vi "insert_log_entry.vi"(8 "error in (no error)":errorcluster, 10 "message":string, 11 "GenericPlugin in":refnum<class "GenericComponent.lvclass">) -> (0 "error out":errorcluster, 3 "GenericPlugin out":refnum<class "GenericComponent.lvclass">)   [LabVIEW 2010, in "GenericComponent.lvclass"]
uses:
  GenericComponent.lvclass
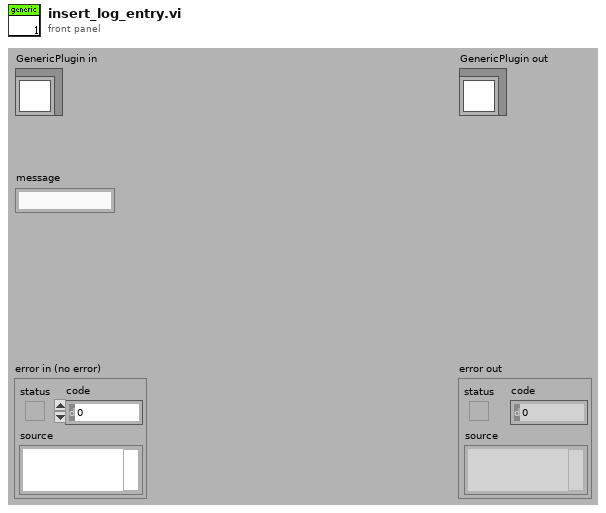
[diagram p1: front panel]
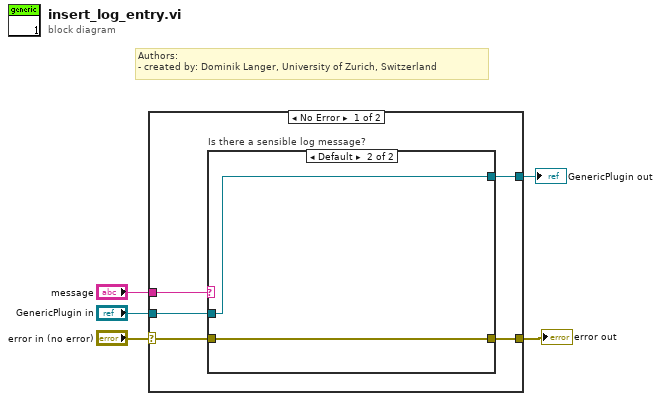
[diagram p0: block diagram]
diagram:
  # "Authors: \n- created by: Dominik Langer, University of Zurich, Switzerland"
  n1 = case shown="No Error" "error in (no error)" {
    selector: "error in (no error)" -> [w10 w16]
    tunnel: [w7 w16] -> w4
    tunnel: [w8 w15] -> w2
    tunnel: "GenericPlugin in" -> [w9 w15]
    tunnel: "message" -> [w6 _]
    frame No Error {
      n2 = case "Is there a sensible log message?" shown="Default" w6 {
        tunnel: w10 -> [w12 w14]
        tunnel: w9 -> [w11 w13]
        tunnel: [w11 w13] -> w8
        tunnel: [w12 w14] -> w7
        frame "" {
        }
        frame Default {
        }
      }
    }
    frame Error {
    }
  }
  "error out" <- w4
  "GenericPlugin out" <- w2
